vi "testing.vi"() -> ()   [LabVIEW 2019]
uses:
  <vilib>/JDP Science/JSONtext/String Subset.vi
  <vilib>/JDP Science/JSONtext/support/Strip Quotes and Unescape.vi
  <vilib>/JDP Science/JSONtext/support/Unescape JSON string.vi
  <vilib>/JDP Science/JSONtext/Parsing/Parse Full Path or Item Name.vi
  <vilib>/JDP Science/JSONtext/Offset/Find Item Locations by Path.vi
  <vilib>/JDP Science/JSONtext/JSONtext.lvlib
panel:
  out "map":map{string, string}(c390)
  in  "Notebook Name":string
  out "Notebook ID":string
  out "key not found?":bool
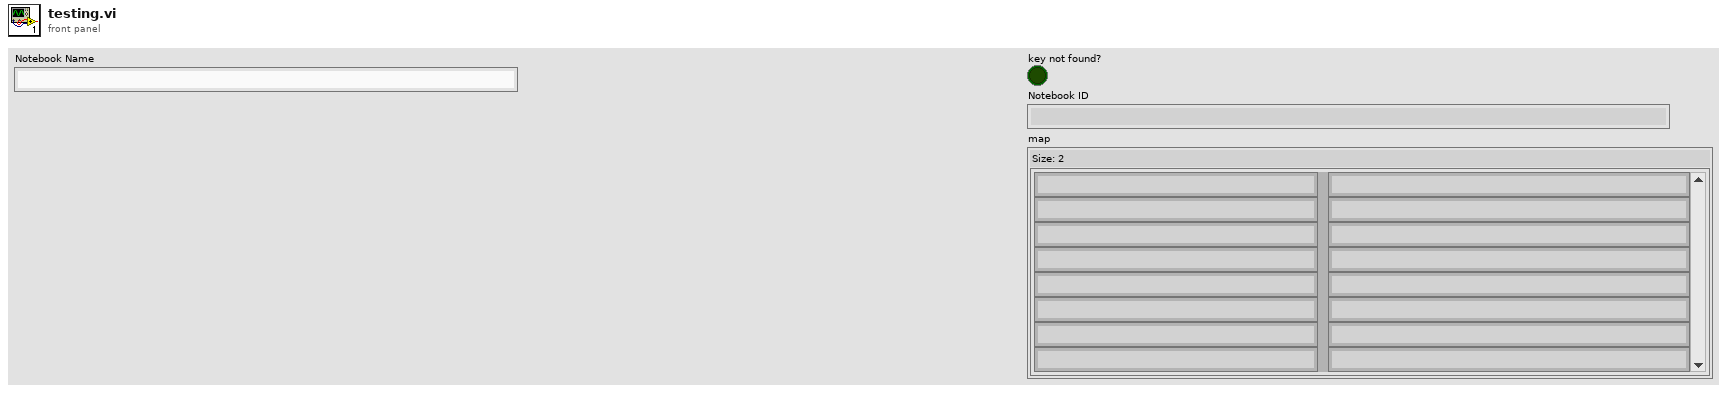
[diagram p1: front panel]
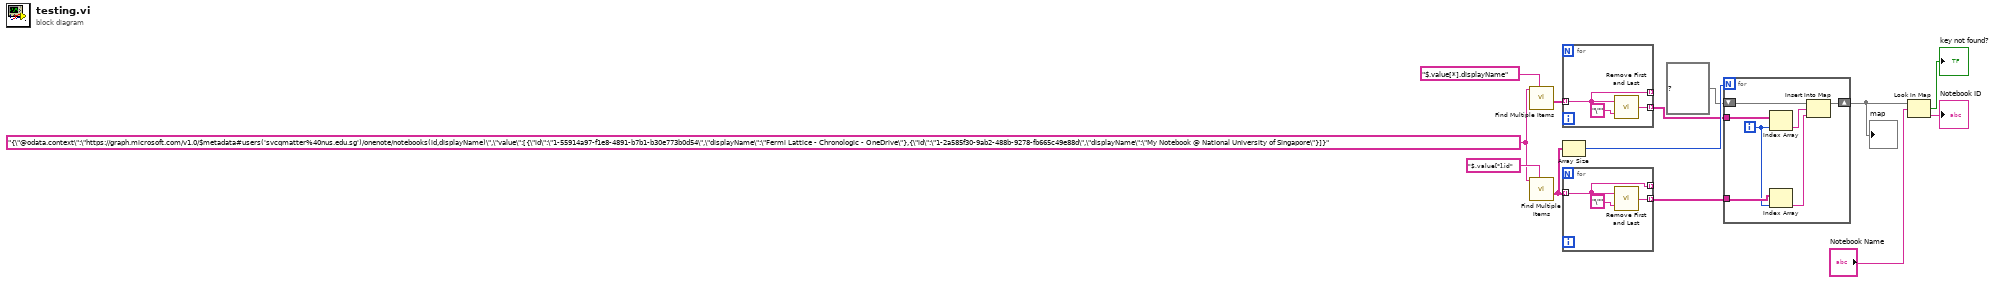
[diagram p0: block diagram]
diagram:
  w11 = "{\"@odata.context\":\"https://graph.microsoft.com/v1.0/$metadata#users('svcqmatter%40nus.edu.sg')/onenote/notebooks(id,displayName)\",\"value\":[{\"id\":\"1-55914a97-f1e8-4891-b7b1-b30e773b0d54\",\"displayName\":\"Fermi Lattice - Chronologic - OneDrive\"},{\"id\":\"1-2a585f30-9ab2-488b-9278-fb665c49e88d\",\"displayName\":\"My Notebook @ National University of Singapore\"}]}"
  n1 = call <vilib>:"Find Multiple Items.vi"("$Path or Item Name"="$.value[*].displayName", "JSON"=w11) -> ("<JSON>"=w9:string[])  [unwired: 6 in, 3 out]
  n2 = call <vilib>:"Find Multiple Items.vi"("$Path or Item Name"="$.value[*].id", "JSON"=w11) -> ("<JSON>"=w12:string[])  [unwired: 6 in, 3 out]
  n3 = for {
    tunnel: w9 -> [w14] mode=indexing
    tunnel: [w14] -> _ mode=indexing
    tunnel: [w15] -> w6 mode=indexing
    n4 = call "Remove First and Last.vi"("Char to Remove"="\"", "String"=w14) -> ("Result"=w15:string)
  }
  n5 = Array Size(array=w12) -> (size(s)=w7:i32)
  n6 = for {
    tunnel: w12 -> [w17] mode=indexing
    tunnel: [w17] -> _ mode=indexing
    tunnel: [w18] -> w8 mode=indexing
    n7 = call "Remove First and Last.vi"("Char to Remove"="\"", "String"=w17) -> ("Result"=w18:string)
  }
  n8 = for {
    N: w7 -> [_]
    tunnel: w8 -> [w26]
    tunnel: w6 -> [w25]
    shift-right: [w22] -> w4
    shift-left: map{string, string} {} ("map") -> [w24]
    i -> [w23]
    n9 = Index Array(array=w25, index=w23) -> (element=w21:string)
    n10 = Index Array(array=w26, index=w23) -> (element=w20:string)
    n11 = Insert Into Map(map in=w24, key=w21, value=w20) -> (map out=w22:map{string, string})  [unwired: 2 out]
  }
  "map" <- w4
  n12 = Look In Map(map=w4, key="Notebook Name") -> (key not found?=→"key not found?":bool, value=→"Notebook ID":string)  [unwired: 1 in]
